vi "test Parse Device Info_2.vi"(11 "Test Case In":refnum<class "test EDS.lvclass">) -> (0 "error out":errorcluster, 3 "Test Case Out":refnum<class "test EDS.lvclass">)   [LabVIEW 2024, in "test EDS.lvclass"]
uses:
  test EDS.lvclass
  test EDS.lvclass/test EDS.ctl
  4993e8ee-a06a-463a-9684-69129f64d5ce.vi
  Core/EDS/EDS.lvclass
  <vilib>/PNR/JSONtext Object Serialization/Generic Object Serializer/Generic Object Serializer.lvclass
  <vilib>/PNR/JSONtext Object Serialization/Generic Object Serializer/Type Name Handling.ctl
  99df47cb-525e-4171-a825-741cf93afc66.vi
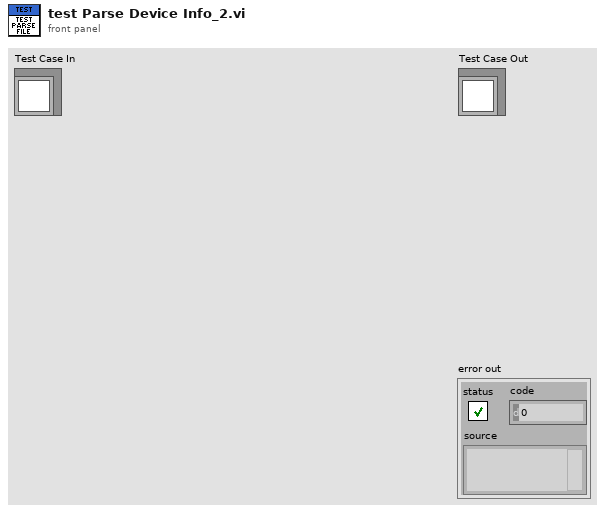
[diagram p1: front panel]
types:
  T1 = typedef "Generic Object Serializer.lvclass/Type Name Handling.ctl" = enum16{"None", "Inline"}
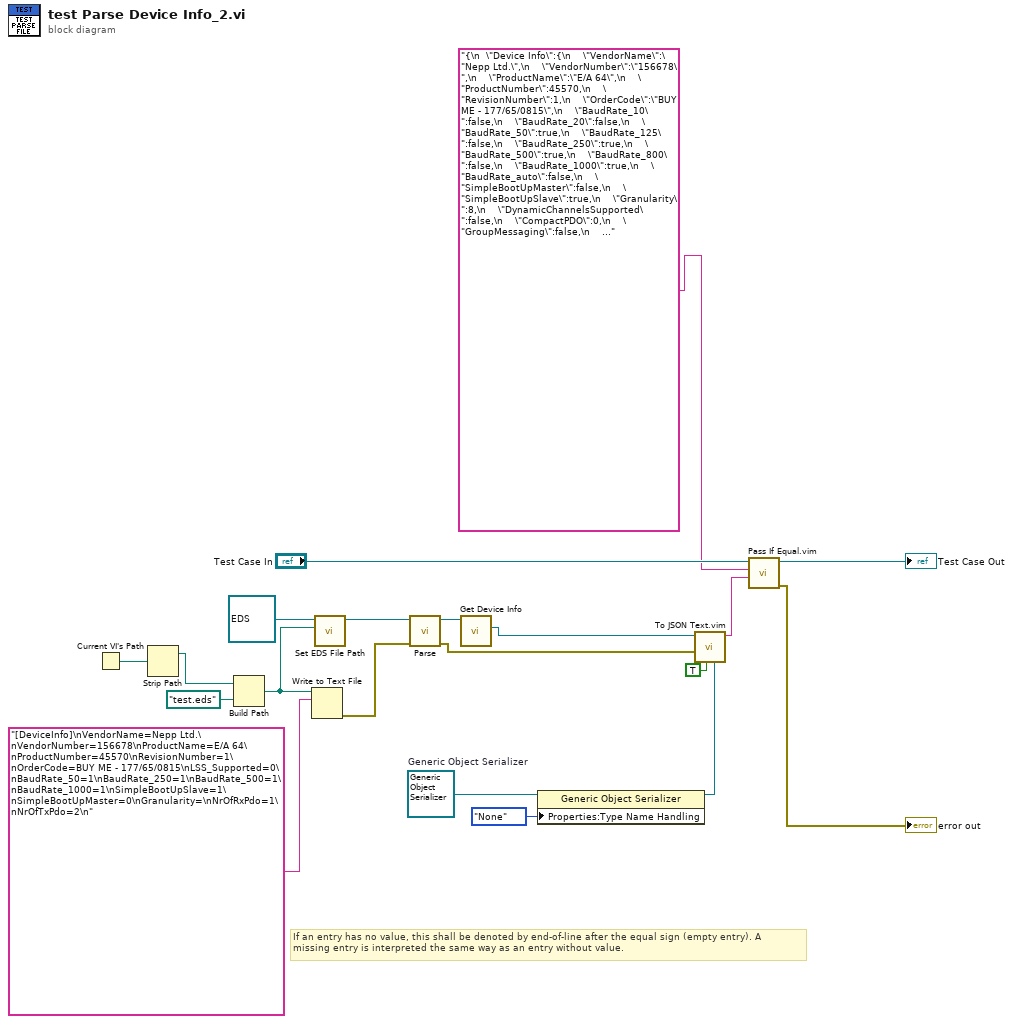
[diagram p0: block diagram]
diagram:
  w7 = refnum<class "Generic Object Serializer.lvclass"> refnum  # Generic Object Serializer
  # "If an entry has no value, this shall be denoted by end-of-line after the equal sign (empty entry). A \nmissing entry is interpreted the same way as an entry without value."
  n1 = Current VI's Path() -> (path=w15:path)
  n2 = Strip Path(path=w15) -> (stripped path=w14:path)  [unwired: 1 out]
  n3 = Build Path(base path=w14, name or relative path=path "test.eds") -> (appended path=w13:path)
  n4 = Write to Text File(file (use dialog)=w13, text="[DeviceInfo]\nVendorName=Nepp Ltd.\nVendorNumber=156678\nProductName=E/A 64\nProductNumber=45570\nRevisionNumber=1\nOrderCode=BUY ME - 177/65/0815\nLSS_Supported=0\nBaudRate_50=1\nBaudRate_250=1\nBaudRate_500=1\nBaudRate_1000=1\nSimpleBootUpSlave=1\nSimpleBootUpMaster=0\nGranularity=\nNrOfRxPdo=1\nNrOfTxPdo=2\n") -> (error out=w11:errorcluster)  [unwired: 2 in, 2 out]
  n5 = call "Set EDS File Path.vi"("EDS File Path"=w13, "EDS in"=refnum<class "EDS.lvclass"> refnum ("EDS.lvlib:EDS.lvclass")) -> ("EDS out"=w16:refnum<class "EDS.lvclass">)  [unwired: 9 in]
  n6 = call "Parse.vi"("error in"=w11, "EDS in"=w16) -> ("error out"=w4:errorcluster, "EDS out"=w9:refnum<class "EDS.lvclass">)  [unwired: 8 in]
  n7 = call "Get Device Info.vi"("EDS in"=w9) -> ("Device Info"=w3:refnum<class "Device Info.lvclass">)  [unwired: 9 in, 1 out]
  n8 = property class="Generic Object Serializer"(reference=w7, "Properties:Type Name Handling"=Type_Name_Handling."None" ("Type Name Handling")) -> (reference out=w6:refnum<class "Generic Object Serializer.lvclass">)  [unwired: 1 in, 1 out]
  n9 = call "To JSON Text.vim"("LVClass Serializer"=w6, "Pretty Print?"=TRUE, "error in (no error)"=w4, "Anything"=w3) -> ("<JSON>"=w1:string)  [unwired: 6 in, 1 out]
  n10 = call "Pass If Equal.vim"("Actual"=w1, "Expected"="{\n  \"Device Info\":{\n    \"VendorName\":\"Nepp Ltd.\",\n    \"VendorNumber\":\"156678\",\n    \"ProductName\":\"E/A 64\",\n    \"ProductNumber\":45570,\n    \"RevisionNumber\":1,\n    \"OrderCode\":\"BUY ME - 177/65/0815\",\n    \"BaudRate_10\":false,\n    \"BaudRate_20\":false,\n    \"BaudRate_50\":true,\n    \"BaudRate_125\":false,\n    \"BaudRate_250\":true,\n    \"BaudRate_500\":true,\n    \"BaudRate_800\":false,\n    \"BaudRate_1000\":true,\n    \"BaudRate_auto\":false,\n    \"SimpleBootUpMaster\":false,\n    \"SimpleBootUpSlave\":true,\n    \"Granularity\":8,\n    \"DynamicChannelsSupported\":false,\n    \"CompactPDO\":0,\n    \"GroupMessaging\":false,\n    \"NrOfRXPDO\":1,\n    \"NrOfTXPDO\":2,\n    \"LSS_Supported\":false,\n    \"LSS_Master\":false,\n    \"NG_Slave\":false,\n    \"NG_Master\":false,\n    \"NrOfNG_MonitoredNodes\":0\n  }\n}" ("<JSON>"), "LUnit Test Case In"="Test Case In") -> ("error out"=→"error out":errorcluster, "LUnit Test Case Out"=→"Test Case Out":refnum<class "test EDS.lvclass">)  [unwired: 7 in]
